vi "StressDist_long_calc.vi"(1 "Angle":dbl, 2 "Parameters":dbl[](array[numeric])) -> (0 "Stress":dbl)   [LabVIEW 2016]
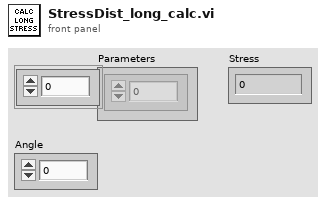
[diagram p1: front panel]
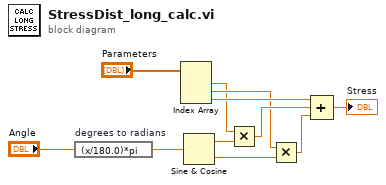
[diagram p0: block diagram]
diagram:
  n1 = expression code="(x/180.0)*pi" "degrees to radians"("Angle") -> (w3:dbl)
  n2 = Index Array(array="Parameters") -> (element #1=w5:dbl, element #2=w7:dbl, element #3=w8:dbl)  [unwired: 3 in]
  n3 = Sine & Cosine(0:w3) -> (1:w4:dbl, 2:w6:dbl)
  n4 = Multiply(x=w5, y=w4) -> (x*y=w9:dbl)
  n5 = Multiply(x=w7, y=w6) -> (x*y=w10:dbl)
  n6 = Compound Arithmetic op=ADD(w8, w9, w10) -> (→"Stress":dbl)
